vi "RubikStop.vi"(8 "error in":errorcluster) -> (0 "error out":errorcluster)   [LabVIEW 2017, in "RubikLibraryRT.lvlib"]
doc: "Put Rubik's solver into end positions:\nAll servos to 0°, all grippers to closed. \n\nInput:\nError in\n\nOutput:\nError out"
uses:
  RubikLibraryRT.lvlib
  ServoEnumControl.ctl
  ServoAbsAngleControl.ctl
  RubikLibrary.lvlib
panel:
  in  "List of Servo Angles":T1[](array[typedef])=[enum."0°", enum."0°", enum."0°"]
  in  "Gripper closed":bool
  in  "List of Servos":T2[](array[typedef])=[enum."Left Servo", enum."Front Servo", enum."Right Servo"]
  # "Rubic Stop"
  # "Rubik Cube Stop Configuration\n\nPosition of Grippers:  Closed\nPosition of Servos: 0°"
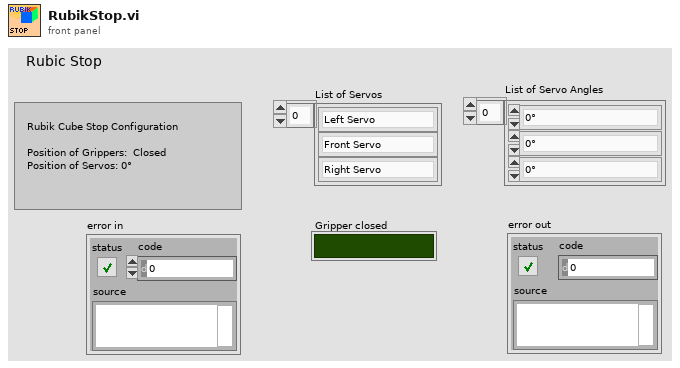
[diagram p1: front panel]
types:
  T1 = typedef "RubikLibrary.lvlib/ServoAbsAngleControl.ctl" = enum16{"+90°", "0°", "-90°"}
  T2 = typedef "RubikLibrary.lvlib/ServoEnumControl.ctl" = enum16{"Left Servo", "Front Servo", "Right Servo"}
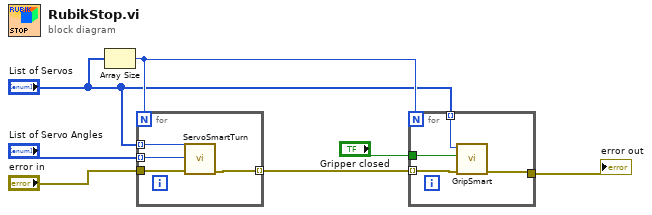
[diagram p0: block diagram]
diagram:
  n1 = Array Size(array="List of Servos") -> (size(s)=w3:i32)
  n2 = for {
    N: w3 -> [_]
    tunnel: "List of Servos" -> [w11] mode=indexing
    tunnel: "List of Servo Angles" -> [w10] mode=indexing
    tunnel: [w9] -> w5 mode=indexing
    tunnel: "error in" -> [w8]
    n3 = call "ServoSmartTurn.vi"("error in"=w8, "Turn to (in)"=w10, "Servo"=w11) -> ("error out"=w9:errorcluster)  [unwired: 7 in, 1 out]
  }
  n4 = for {
    N: w3 -> [_]
    tunnel: [w15] -> w4
    tunnel: "Gripper closed" -> [w14]
    tunnel: "List of Servos" -> [w13] mode=indexing
    tunnel: w5 -> [w12] mode=indexing
    n5 = call "GripSmart.vi"("error in"=w12, "Grip closed (in)"=w14, "Servo"=w13) -> ("error out"=w15:errorcluster)  [unwired: 7 in, 1 out]
  }
  "error out" <- w4
